vi "CRYPEAQ WOME.vi"(11 "f":dbl[](array[numeric])) -> (3 "W2":dbl[](array[numeric]))   [LabVIEW 2013]
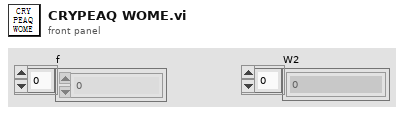
[diagram p1: front panel]
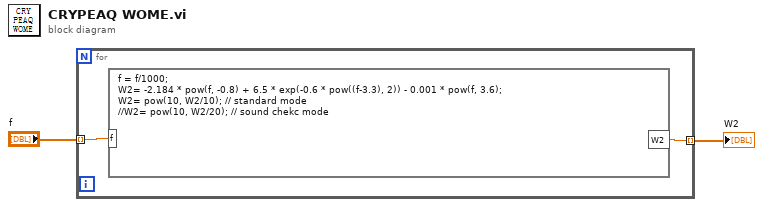
[diagram p0: block diagram]
diagram:
  n1 = for {
    tunnel: "f" -> [w4] mode=indexing
    tunnel: [w3] -> w1 mode=indexing
    n2 = formula code="f = f/1000; \nW2= -2.184 * pow(f, -0.8) + 6.5 * exp(-0.6 * pow((f-3.3), 2)) - 0.001 * pow(f, 3.6);\nW2= pow(10, W2/10); // standard mode\n//W2= pow(10, W2/20); // sound chekc mode"("f"=w4) -> ("W2"=w3:dbl)
  }
  "W2" <- w1
